vi "Move Window to Top (hwnd).vi"(8 "error in (no error)":errorcluster, 9 "Activate? (F)":bool, 10 "Window Name (\"\")":string, 11 "HWnd":u32) -> (0 "error out":errorcluster, 3 "HWnd Out":u32)   [LabVIEW 2011]
doc: "This function will make the window named in the 'window name' input, or identified by the 'window refnum' the top window, and activate it (default case). If 'not a window refnum' is passed in, then the function will use the window name to get a window window refnum. If the window cannot be found, an error will be returned.\n\n-------------\nDeveloped by Brian Hoover (hooovahh)"
uses:
  <userlib>/_OpenG.lib/error/error.llb/Build Error Cluster__ogtk.vi
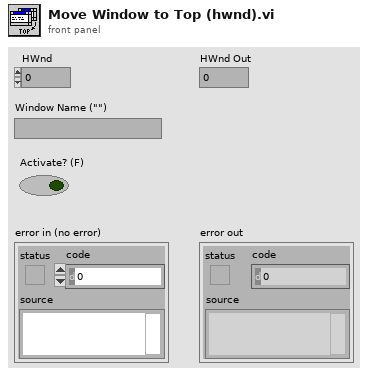
[diagram p1: front panel]
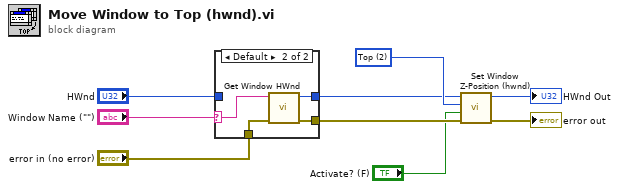
[diagram p0: block diagram]
diagram:
  w6 = i16 2 items=["Not Topmost", "Topmost", "Top", "Bottom"]
  n1 = case shown="Default" "Window Name (\"\")" {
    selector: "Window Name (\"\")" -> [_ w12]
    tunnel: "error in (no error)" -> [w10 w15]
    tunnel: [w11 w14] -> w5
    tunnel: "HWnd" -> [w11 _]
    tunnel: [w10 w13] -> w4
    frame "" {
    }
    frame Default {
      n2 = call "Get Window HWnd.vi"("error in (no error)"=w15, "Window Name"=w12) -> ("error out"=w13:errorcluster, "HWnd Out"=w14:u32)  [unwired: 8 in]
    }
  }
  n3 = call "Set Window Z-Position (hwnd).vi"("error in (no error)"=w4, "Activate? (F)"="Activate? (F)", "Z-Order Position"=w6, "HWnd"=w5) -> ("error out"=→"error out":errorcluster, "HWnd Out"=→"HWnd Out":u32)  [unwired: 6 in]
